vi "TD3_CalculatriceSimple.vi"() -> ()   [LabVIEW 2015]
panel:
  out "Courant":dbl
  out "Indice de la touche":i32
  out "?":bool[](array[boolean])
  out "Résultat":dbl
  in  "?":T1
  in  "?":bool
  # "Calculatrice"
  # "0     1     2     3    4     5     6     7     8     9     +     -      *     /      R     =    C"
  # "C"
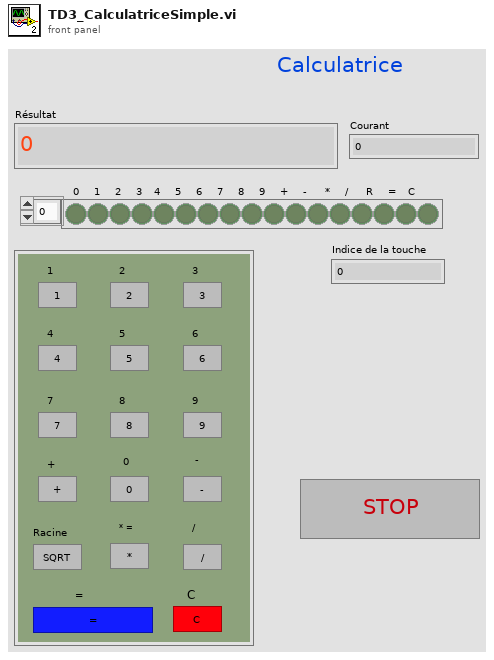
[diagram p1: front panel]
types:
  T1 = cluster{" 0      ":bool, "   1":bool, "   2":bool, "   3":bool, "   4":bool, "   5":bool, "   6":bool, "   7":bool, "   8":bool, "   9":bool, "   +":bool, "    -":bool, "   * =":bool, "   /":bool, "Racine":bool, "            =":bool, bool}
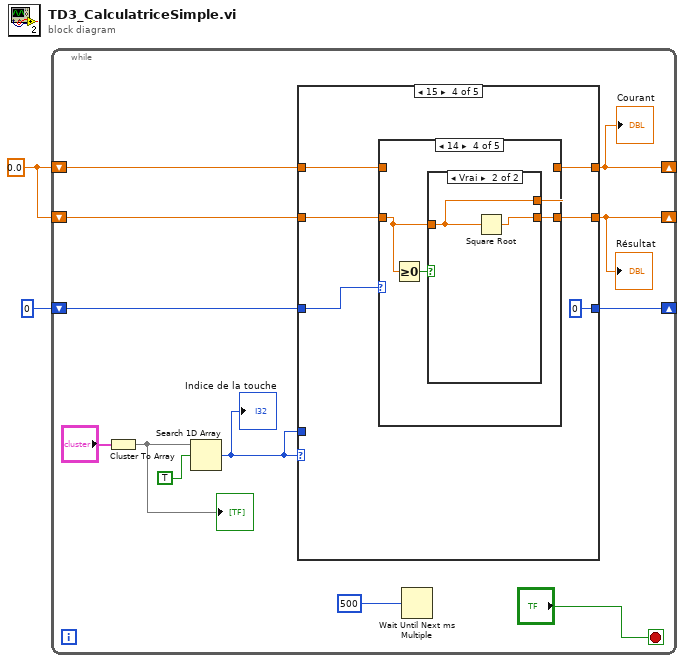
[diagram p0: block diagram]
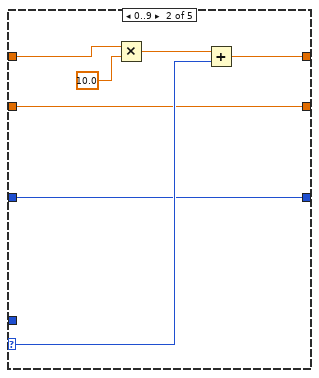
[diagram p3: hidden frame]
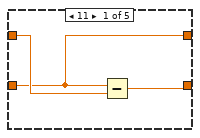
[diagram p5: hidden frame]
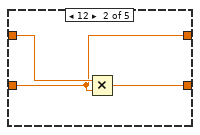
[diagram p6: hidden frame]
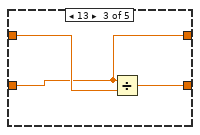
[diagram p7: hidden frame]
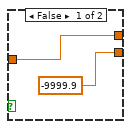
[diagram p8: hidden frame]
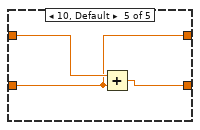
[diagram p9: hidden frame]
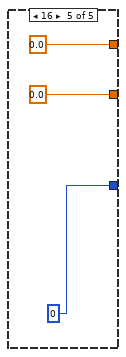
[diagram p10: hidden frame]
diagram:
  w2 = 0.0
  n1 = while {
    shift-right: [w7] -> _
    shift-left: w2 -> [w10]
    shift-right: [w8] -> _
    shift-left: w2 -> [w9]
    shift-right: [w4] -> _
    shift-left: 0 -> [w6]
    stop <- "?" stop-if-true
    n2 = Cluster To Array(cluster="?") -> (array=w3:bool[])
    "?" <- w3
    n3 = Search 1D Array(1D array=w3, element=TRUE) -> (index of element=w5:i32)  [unwired: 1 in]
    "Indice de la touche" <- w5
    n4 = case shown="15" w5 {
      selector: w5 -> [_ w21 _ _ _]
      tunnel: w10 -> [w17 w24 w26 w33 _]
      tunnel: [w17 w20 w27 w30 0.0] -> w7
      tunnel: w9 -> [w16 w19 w27 w32 _]
      tunnel: [w16 w19 w26 w31 0.0] -> w8
      tunnel: w6 -> [w15 w18 _ w29 _]
      tunnel: w5 -> [_ _ w25 _ _]
      tunnel: [w15 w18 w25 0 0] -> w4
      frame -1, Default {
      }
      frame 0..9 {
        n5 = Multiply(x=w24, y=10.0) -> (x*y=w22:dbl)
        n6 = Add(x=w22, y=w21) -> (x+y=w20:dbl)
      }
      frame 10..14 {
      }
      frame 15 {
        n7 = case shown="14" w29 {
          tunnel: w33 -> [w35 w38 w41 _ w53]
          tunnel: w32 -> [w34 w37 w40 w43 w51]
          tunnel: [w36 w39 w42 w45 w52] -> w31
          tunnel: [w34 w37 w40 w44 w51] -> w30
          frame 11 {
            n8 = Subtract(x=w34, y=w35) -> (x-y=w36:dbl)
          }
          frame 12 {
            n9 = Multiply(x=w38, y=w37) -> (x*y=w39:dbl)
          }
          frame 13 {
            n10 = Divide(x=w40, y=w41) -> (x/y=w42:dbl)
          }
          frame 14 {
            n11 = Greater Or Equal To 0?(x=w43) -> (x >= 0?=w46:bool)
            n12 = case shown="Vrai" w46 {
              tunnel: [-9999.9 w50] -> w45
              tunnel: w43 -> [w48 w49]
              tunnel: [w48 w49] -> w44
              frame False {
              }
              frame True {
                n13 = Square Root(x=w49) -> (sqrt(x)=w50:dbl)
              }
            }
          }
          frame 10, Default {
            n14 = Add(x=w53, y=w51) -> (x+y=w52:dbl)
          }
        }
      }
      frame 16 {
      }
    }
    "Résultat" <- w8
    "Courant" <- w7
    n15 = Wait Until Next ms Multiple(millisecond multiple=u32 500) -> ()  [unwired: 1 out]
  }
